vi "Control Events.vi"(8 "error in (no error)":errorcluster, 11 "ButtonControl in":refnum<class "DigitalButtonControl.lvclass">) -> (0 "error out":errorcluster, 2 "Control Events":refnum<class "Control Event Registrations.lvclass">, 3 "ButtonControl out":refnum<class "DigitalButtonControl.lvclass">)   [LabVIEW 2020, in "VolatusGUIElements.lvlib" / "DigitalButtonControl.lvclass"]
uses:
  DigitalButtonControl.lvclass
  VolatusGUI/Control Event Registrations/Control Event Registrations.lvclass
  DigitalButtonControl.lvclass/DigitalButtonControl.ctl
  C:/dev/lv20CE/relink/lv-volatus/VolatusGUI/Control/Control.lvclass
  C:/dev/lv20CE/relink/lv-volatus/VolatusGUI/GUI Element/GUI Element.lvclass
  C:/dev/lv20CE/relink/lv-volatus/VolatusGUIElements/DigitalButtonControl/DigitalButtonControl.lvclass
  C:/dev/lv20CE/relink/lv-volatus/VolatusGUI/OnValueChangeHandler/OnValueChangeHandler.lvclass
  VolatusGUI/GUI Element/GUI Element.lvclass
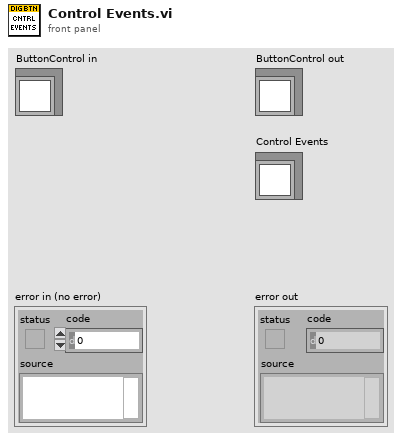
[diagram p1: front panel]
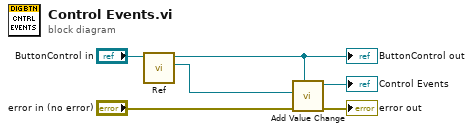
[diagram p0: block diagram]
diagram:
  n1 = call "Ref.vi"("GUI Element in"="ButtonControl in") -> ("Ref"=w3:refnum<vi>, "GUI Element out"=w4:refnum<class "DigitalButtonControl.lvclass">)  [unwired: 9 in]
  "ButtonControl out" <- w4
  n2 = call "Add Value Change.vi"("Control"=w4, "error in (no error)"="error in (no error)", "CtlRef"=w3) -> ("error out"=→"error out":errorcluster, "Control Event Registrations out"=→"Control Events":refnum<class "Control Event Registrations.lvclass">)  [unwired: 7 in]
